vi "Simulate Hadware.vi"(8 "error in":errorcluster) -> (0 "error out":errorcluster)   [LabVIEW 2025, in "Runtime Configuration Support Example Engine.lvlib"]
uses:
  Runtime Configuration Support Example Engine.lvlib
  HW Operations.ctl
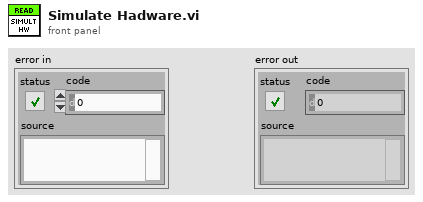
[diagram p1: front panel]
types:
  T1 = typedef "HW Operations.ctl" = enum16{"Initialize", "Set In Val", "Get In Val", "Set Block", "Set Out Val", "Get Out Val", "Get In Array", "Get Out Array"}
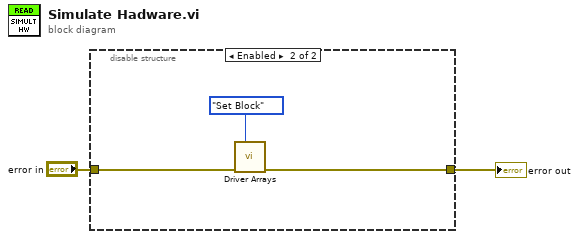
[diagram p0: block diagram]
diagram:
  n1 = disable-structure shown="Enabled" {
    disable-tunnel: [w3 w4] -> w2
    disable-tunnel: "error in" -> [w3 w5]
    frame Disabled {
    }
    frame Enabled {
      n2 = call "Driver Arrays.vi"("error in"=w5, "Curr Operation"=HW_Operations."Set Block") -> ("error out"=w4:errorcluster)  [unwired: 6 in, 3 out]
    }
  }
  "error out" <- w2
